vi "get center freq.vi"(8 "error in (no error)":errorcluster) -> (0 "error out":errorcluster)   [LabVIEW 2013, in "rtlsdr.lvlib"]
doc: "RTLSDR_API uint32_t rtlsdr_get_center_freq(rtlsdr_dev_t *dev);"
uses:
  rtlsdr.lvlib
  rtlsdr.dll
panel:
  out "dev 2":u64
  out "center_freq":u32
  in  "dev":u64
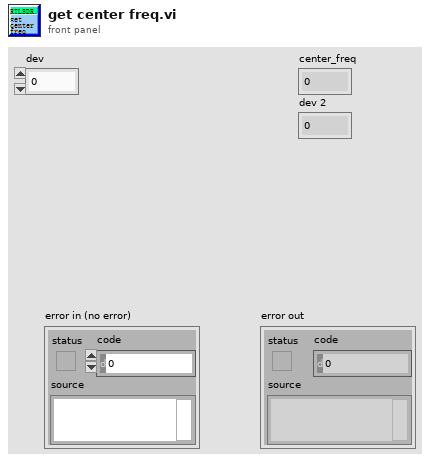
[diagram p1: front panel]
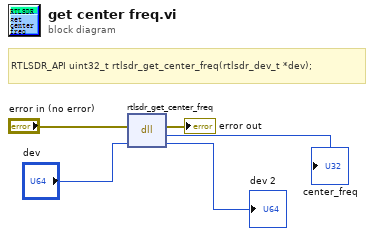
[diagram p0: block diagram]
diagram:
  # "RTLSDR_API uint32_t rtlsdr_get_center_freq(rtlsdr_dev_t *dev);"
  n1 = dll-call lib="D:/SDRDriver/Lab1/rtlsdr.*" fn="rtlsdr_get_center_freq"(error in="error in (no error)", "dev"="dev") -> (error out=→"error out":errorcluster, "center_freq"=→"center_freq":u32, "dev"=→"dev 2":u64)  [unwired: 2 in, 1 out]
